vi "FTW-ScripterStep-Base_ScripterInbox_Get.vi"(8 "error in (no error)":errorcluster, 11 "FTW-ScripterStep-Base in":refnum<class "FTW-ScripterStep-Base.lvclass">) -> (0 "error out":errorcluster, 2 "Scripter Inbox":string, 3 "FTW-ScripterStep-Base out":refnum<class "FTW-ScripterStep-Base.lvclass">)   [LabVIEW 2015, in "FTW-ScripterStep-Base.lvclass"]
uses:
  FTW-ScripterStep-Base.lvclass
  FTW-ScripterStep-Base.lvclass/FTW-ScripterStep-Base.ctl
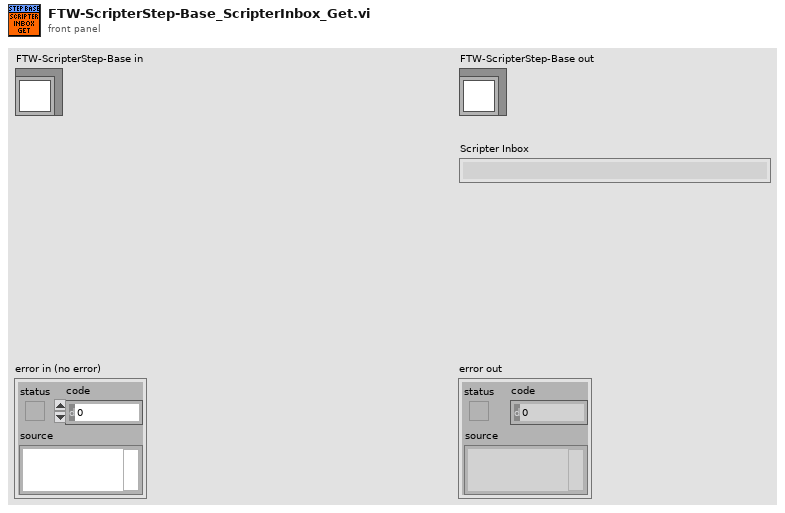
[diagram p1: front panel]
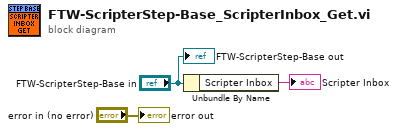
[diagram p0: block diagram]
diagram:
  n1 = Unbundle By Name("FTW-ScripterStep-Base in") -> ("Scripter Inbox"=→"Scripter Inbox":string)
  "error out" <- "error in (no error)"
  "FTW-ScripterStep-Base out" <- "FTW-ScripterStep-Base in"
